vi "MTMount_getSample_LockingPins.vi"(8 "error in (no error)":errorcluster, 11 "Locking_Pins_Ctl":T1) -> (0 "error out":errorcluster, 2 "function return":i32, 3 "Locking_Pins_Ctl out":T1)   [LabVIEW 2018, in "SALLV_MTMount.lvlib"]
doc: "int MTMount_shm_getSample_Locking_PinsLV(MTMount_Locking_PinsLV *Locking_Pins_Ctl );"
uses:
  SALLV_MTMount.lvlib
  DataTypes/Locking_Pins.ctl
  SALLV_MTMount.so
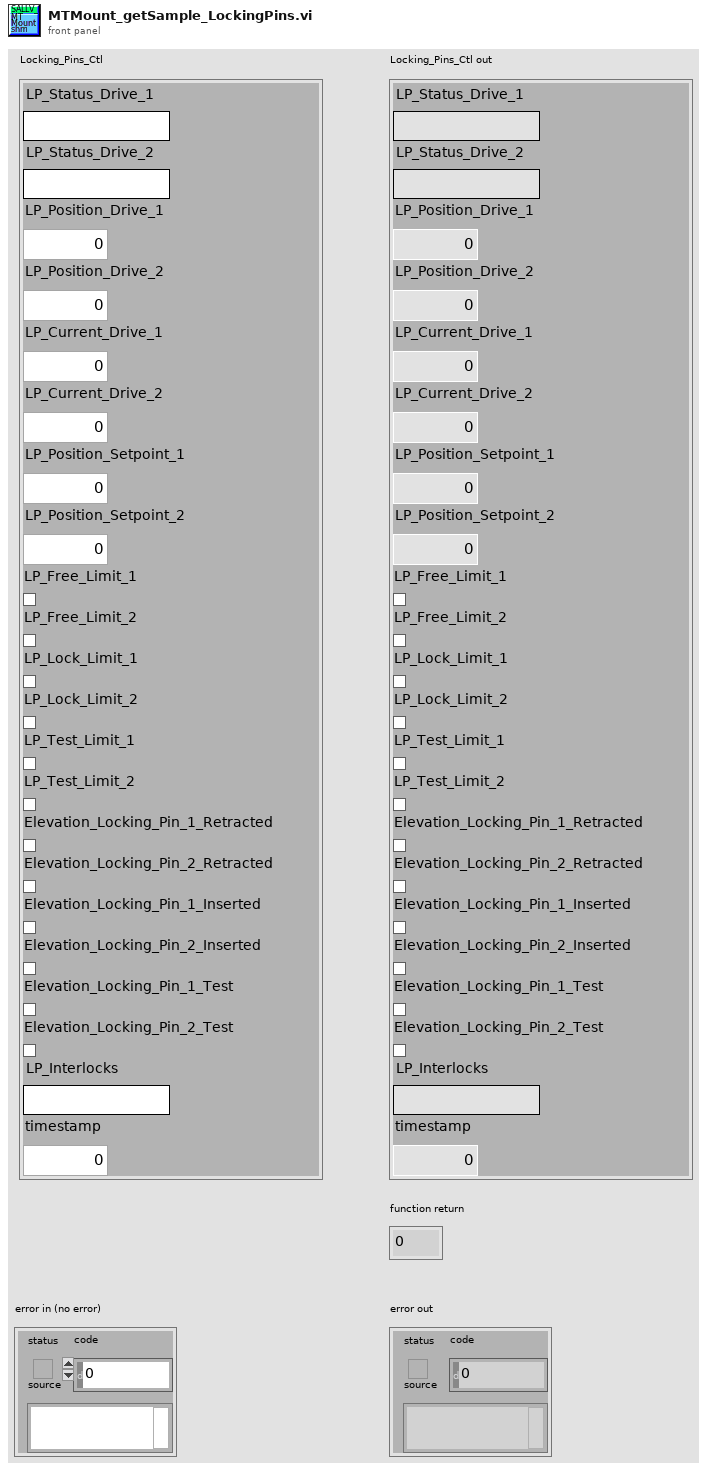
[diagram p1: front panel]
types:
  T1 = typedef "SALLV_MTMount.lvlib/Locking_Pins.ctl" = cluster{"LP_Status_Drive_1":string, "LP_Status_Drive_2":string, "LP_Position_Drive_1":dbl, "LP_Position_Drive_2":dbl, "LP_Current_Drive_1":dbl, "LP_Current_Drive_2":dbl, "LP_Position_Setpoint_1":dbl, "LP_Position_Setpoint_2":dbl, "LP_Free_Limit_1":bool, "LP_Free_Limit_2":bool, "LP_Lock_Limit_1":bool, "LP_Lock_Limit_2":bool, "LP_Test_Limit_1":bool, "LP_Test_Limit_2":bool, "Elevation_Locking_Pin_1_Retracted":bool, "Elevation_Locking_Pin_2_Retracted":bool, "Elevation_Locking_Pin_1_Inserted":bool, "Elevation_Locking_Pin_2_Inserted":bool, "Elevation_Locking_Pin_1_Test":bool, "Elevation_Locking_Pin_2_Test":bool, "LP_Interlocks":string, "timestamp":dbl}
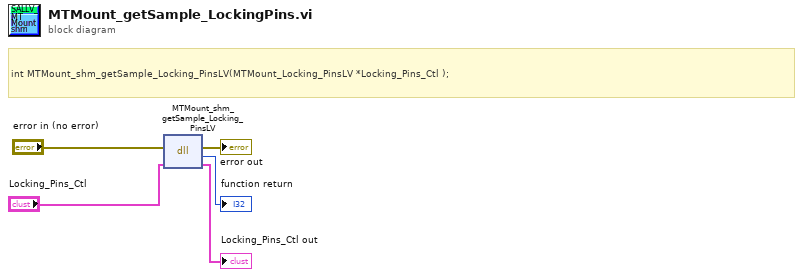
[diagram p0: block diagram]
diagram:
  # "int MTMount_shm_getSample_Locking_PinsLV(MTMount_Locking_PinsLV *Locking_Pins_Ctl );"
  n1 = dll-call lib="home/ttsai/Document/salApiMTMount/SALLV_MTMount/SALLV_MTMount.*" fn="MTMount_shm_getSample_Locking_PinsLV"(error in="error in (no error)", "Locking_Pins_Ctl"="Locking_Pins_Ctl") -> (error out=→"error out":errorcluster, →"function return":i32, "Locking_Pins_Ctl"=→"Locking_Pins_Ctl out":T1)  [unwired: 2 in, 1 out]
